vi "Meas Result Generate TWM Digitizer Correction - fit Gain Phase.vi"(7 "use time shift (true)":bool=TRUE, 9 "phase [rad]":dbl[](array[numeric]), 10 "gain [V/V]":dbl[](array[numeric]), 11 "f [Hz]":dbl[](array[numeric])) -> (0 "time shift [s]":dbl, 1 "DC gain":dbl, 2 "phase out [rad]":dbl[](array[numeric]), 3 "gain out [V/V]":dbl[](array[numeric]))   [LabVIEW 2020]
uses:
  <vilib>/Analysis/baseanly.llb/Mean (DBL).vi
  <vilib>/Analysis/NI_AALBase.lvlib
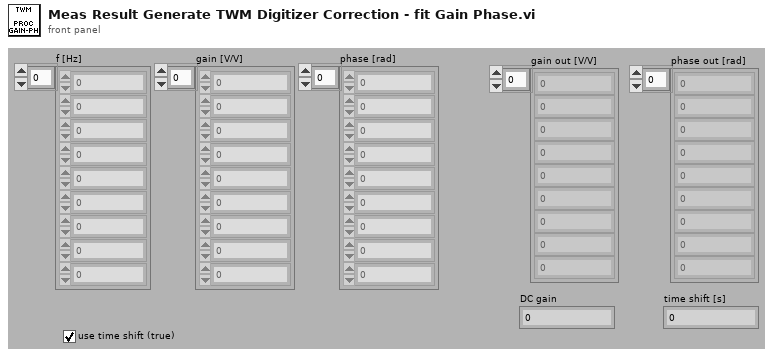
[diagram p1: front panel]
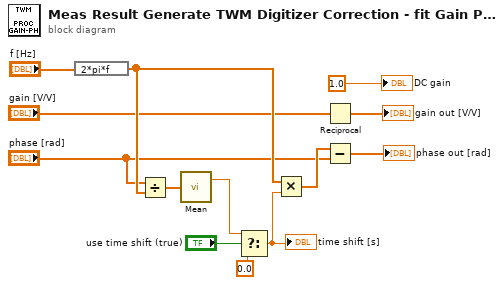
[diagram p0: block diagram]
diagram:
  n1 = expression code="2*pi*f"("f [Hz]") -> (w8:dbl[])
  n2 = Divide(x="phase [rad]", y=w8) -> (x/y=w12:dbl[])
  n3 = call-poly <vilib>:"Mean.vi"("X"=w12) -> ("mean"=w10:dbl)  [unwired: 1 out]
  n4 = Select(t=w10, s="use time shift (true)", f=0.0) -> (s? t:f=w6:dbl)
  "time shift [s]" <- w6
  n5 = Multiply(x=w8, y=w6) -> (x*y=w2:dbl[])
  n6 = Reciprocal(x="gain [V/V]") -> (1/x=→"gain out [V/V]":dbl[])
  n7 = Subtract(x=w2, y="phase [rad]") -> (x-y=→"phase out [rad]":dbl[])
  "DC gain" <- 1.0 ("DC gain")
